vi "Code Point Is Equal To.vi"(2 "Code Point":u32, 3 "Tokenizer":T1) -> (0 "Code Point Equals?":bool)   [LabVIEW 2020, in "Stream.lvlib" / "URLPattern.lvclass"]
uses:
  URLPattern.lvclass
  Tokenizer.ctl
  Tokenize Policy.ctl
  Token.ctl
  Token Type.ctl
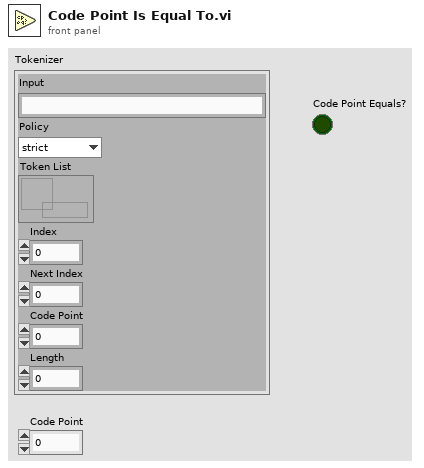
[diagram p1: front panel]
types:
  T1 = typedef "Stream.lvlib/URLPattern.lvclass/Tokenizer.ctl" = cluster{"Input":string, "Policy":T2, "Token List":refnum<queue>, "Index":i32, "Next Index":i32, "Code Point":u32, "Length":i32}
  T2 = typedef "Stream.lvlib/URLPattern.lvclass/Tokenize Policy.ctl" = enum16{"strict", "lenient"}
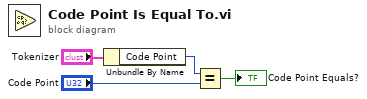
[diagram p0: block diagram]
diagram:
  n1 = Unbundle By Name("Tokenizer") -> ("Code Point"=w3:u32)
  n2 = Equal?(x=w3, y="Code Point") -> (x = y?=→"Code Point Equals?":bool)
